vi "Configure Device Group.vi"(8 "error in (no error)":errorcluster, 10 "Device Group (\"DEFAULT\")":string="DEFAULT", 11 "VISA resource name":refnum<visa-resource-name>) -> (0 "error out":errorcluster, 3 "VISA resource name out":refnum<visa-resource-name>)   [LabVIEW 2020, in "Rohde&Schwarz CMXP Base.lvlib"]
doc: "Sets the \"Device Group\" that the instrument belongs to. For remote installation, this setting must match the corresponding setting in the R&S Software Distributor options.\n\nAttribute:\nRSCMXPBASE_ATTR_DEVICE_GROUP\n\nRemote-control command:\nSYSTem:UPDate:DGRoup"
uses:
  <instrlib>/Rohde&Schwarz CMXP Base/Rohde&Schwarz CMXP Base.lvlib
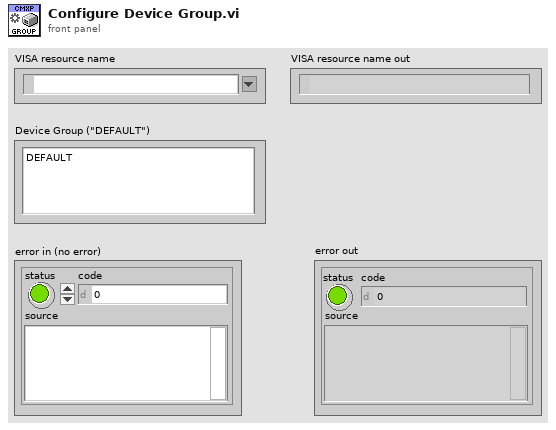
[diagram p1: front panel]
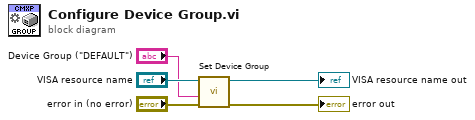
[diagram p0: block diagram]
diagram:
  n1 = call "Set Device Group"("error in (no error)"="error in (no error)", "Device Group ()"="Device Group (\"DEFAULT\")", "instrument handle"="VISA resource name") -> ("error out"=→"error out":errorcluster, "instrument handle out"=→"VISA resource name out":refnum<visa-resource-name>)  [unwired: 7 in]
